vi "H.Signal.vi"() -> (4 "Slide servo home RS":bool, 6 "H.Signal":T2, 8 "LCD Pressing servo home RS":bool, 10 "Error Message":string, 13 "Camera & LVDT cyl":T1, 15 "Bool_H Sig":bool)   [LabVIEW 2020]
uses:
  Galobal variable_TI.vi
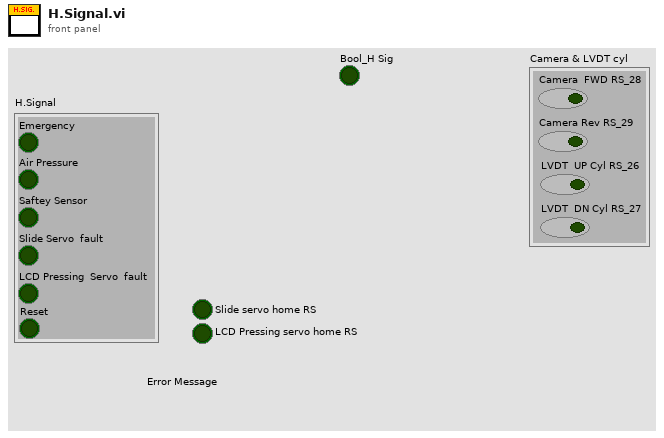
[diagram p1: front panel]
types:
  T1 = cluster{"Camera  FWD RS_28":bool, "Camera Rev RS_29":bool, "LVDT  UP Cyl RS_26":bool, "LVDT  DN Cyl RS_27":bool}
  T2 = cluster{"Emergency":bool, "Air Pressure":bool, "Saftey Sensor":bool, "Slide Servo  fault":bool, "LCD Pressing  Servo  fault":bool, "Reset":bool}
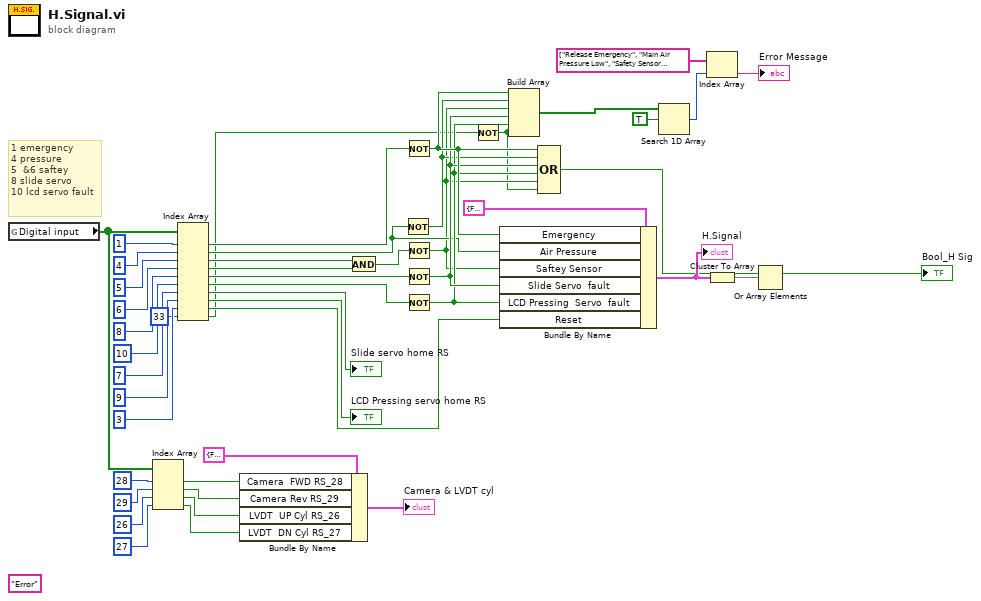
[diagram p0: block diagram]
diagram:
  (unwired) "Error" ("string")
  # "1 emergency\n4 pressure\n5  &6 saftey\n8 slide servo\n10 lcd servo fault"
  n1 = global read "Galobal variable_TI.vi" "Digital input"() -> (w14:bool[])
  n2 = Index Array(array=w14, index #1=28 ("index"), index #2=29 ("index"), index #3=26 ("index"), index #4=27 ("index")) -> (element #1=w10:bool, element #2=w9:bool, element #3=w6:bool, element #4=w5:bool)
  n3 = Index Array(array=w14, index #1=1 ("index"), index #2=4 ("index"), index #3=5 ("index"), index #4=6 ("index"), index #5=8 ("index"), index #6=10 ("index"), index #7=7 ("index"), index #8=9 ("index"), index #9=3 ("index"), index #10=33 ("index")) -> (element #1=w25:bool, element #2=w17:bool, element #3=w41:bool, element #4=w40:bool, element #5=w23:bool, element #6=w22:bool, element #7=→"Slide servo home RS":bool, element #8=→"LCD Pressing servo home RS":bool, element #9=w26:bool, element #10=w2:bool)
  n4 = Bundle By Name(cluster=T1 {"Camera  FWD RS_28"=FALSE, "Camera Rev RS_29"=FALSE, "LVDT  UP Cyl RS_26"=FALSE, "LVDT  DN Cyl RS_27"=FALSE} ("Camera & LVDT cyl"), "Camera  FWD RS_28"=w10, "Camera Rev RS_29"=w9, "LVDT  UP Cyl RS_26"=w6, "LVDT  DN Cyl RS_27"=w5) -> (→"Camera & LVDT cyl":T1)
  n5 = And(x=w41, y=w40) -> (x .and. y?=w24:bool)
  n6 = Not(x=w17) -> (.not. x?=w16:bool)
  n7 = Not(x=w25) -> (.not. x?=w20:bool)
  n8 = Not(x=w24) -> (.not. x?=w15:bool)
  n9 = Not(x=w23) -> (.not. x?=w19:bool)
  n10 = Not(x=w22) -> (.not. x?=w18:bool)
  n11 = Not(x=w2) -> (.not. x?=w1:bool)
  n12 = Bundle By Name(cluster=T2 {"Emergency"=FALSE, "Air Pressure"=FALSE, "Saftey Sensor"=FALSE, "Slide Servo  fault"=FALSE, "LCD Pressing  Servo  fault"=FALSE, "Reset"=FALSE} ("Cluster"), "Emergency"=w20, "Air Pressure"=w17, "Saftey Sensor"=w15, "Slide Servo  fault"=w19, "LCD Pressing  Servo  fault"=w18, "Reset"=w26) -> (w31:T2)
  "H.Signal" <- w31
  n13 = Build Array(w20, w16, w15, w19, w18, w1) -> (w36:bool[])
  n14 = Compound Arithmetic op=OR(w20, w16, w19, w18, w15, w1) -> (→"Bool_H Sig":bool)
  n15 = Search 1D Array(1D array=w36, element=TRUE) -> (index of element=w38:i32)  [unwired: 1 in]
  n16 = Index Array(array=string[] ["Release Emergency", "Main Air Pressure Low", "Safety Sensor Disturb", "Fixture Slide Servo Fault", "LCD Pressing Servo Fault", "Fixture is clamp. Press Home Button "], index=w38) -> (element=→"Error Message":string)
  n17 = Cluster To Array(cluster=w31) -> (array=w30:bool[])
  n18 = Or Array Elements(Boolean array=w30) -> ()  [unwired: 1 out]
